vi "CallBack.vi"(4 "识别结果":refnum<vi>, 5 "事件数据":cluster{"sender":refnum<k24>, "e":refnum<k24>}, 6 "控件引用":refnum<k24>, 7 "事件通用数据":cluster{"事件源":i32, "事件类型":u32, "时间标识":u32}) -> ()   [LabVIEW 2023]
uses:
  System.Speech
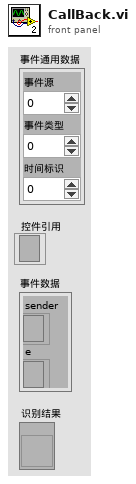
[diagram p1: front panel]
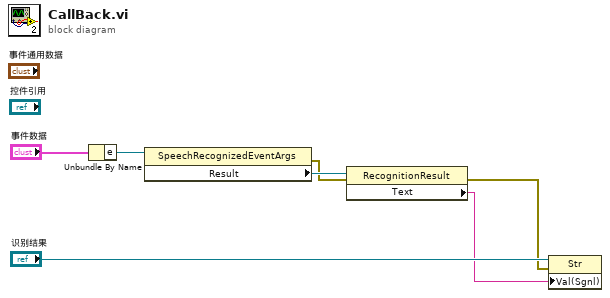
[diagram p0: block diagram]
diagram:
  n1 = Unbundle By Name("事件数据") -> ("e"=w6:refnum<k24>)
  n2 = property class="SpeechRecognizedEventArgs"(reference=w6) -> (error out=w4:errorcluster, "Result"=w5:refnum<k24>)  [unwired: 1 in, 1 out]
  n3 = property class="RecognitionResult"(reference=w5, error in=w4) -> (error out=w1:errorcluster, "Text"=w2:string)  [unwired: 1 out]
  n4 = property class="Str"(reference="识别结果", error in=w1, "Val(Sgnl)"=w2) -> ()  [unwired: 2 out]
